vi "AWS Keys Updater(SubVI).vi"(7 "Queue in":refnum<queue>, 8 "error in (no error)":errorcluster) -> ()   [LabVIEW 2019]
doc: "Updates the AWS Access and Secret keys if a properly formatted file is received in the ~/AWS/incoming folder. \n\nThis is to do on-the-fly changes to the AWS credentials (without stopping/restarting MODAQ) and is not a subsitution to valid keys being set in the configurator.\n\nWhy is this necessary? For security purposes, some organizations may time limit AWS keys. It's possible that the AWS keys could expire during a long MODAQ deployment, therefore we provide a way to hot-update the AWS keys without stopping the current MODAQ run. \n\n2021 NREL"
uses:
  Globals and Definitions/System Message.ctl
  Globals and Definitions/Initialization Globals.vi
  Globals and Definitions/RT Globals RD v1.0.vi
  <vilib>/National Instruments/LabVIEW Interface for Amazon S3/LV Interface for Amazon S3.lvlib
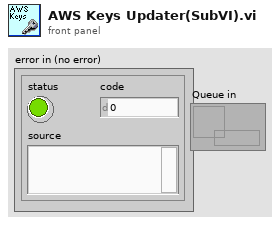
[diagram p1: front panel]
types:
  T1 = typedef "System Message.ctl" = cluster{"Message Tag":string, "Message Body":string, "Snooze Time (s)":dbl, "Snooze Alert?":bool, "Log Event?":bool, "Send Email":i32}
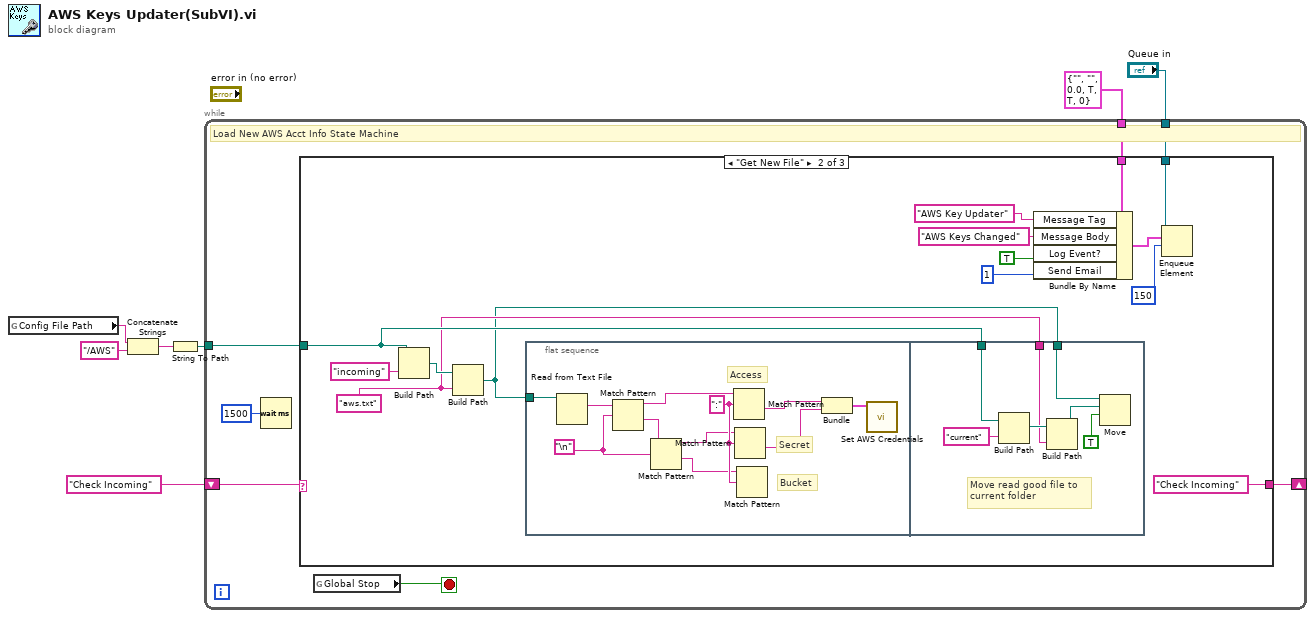
[diagram p0: block diagram]
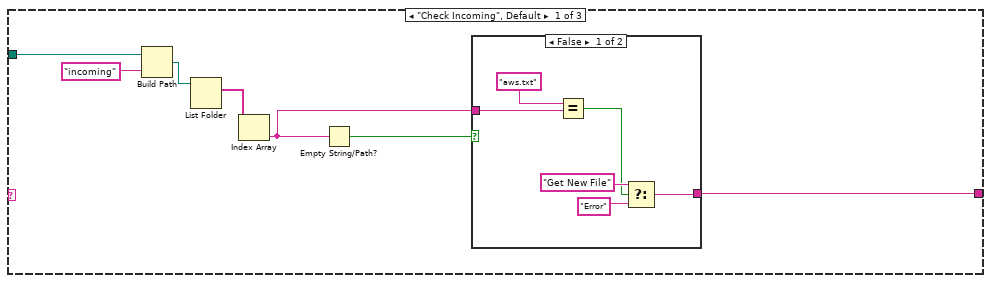
[diagram p2: hidden frame]
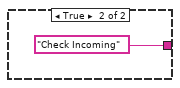
[diagram p3: hidden frame]
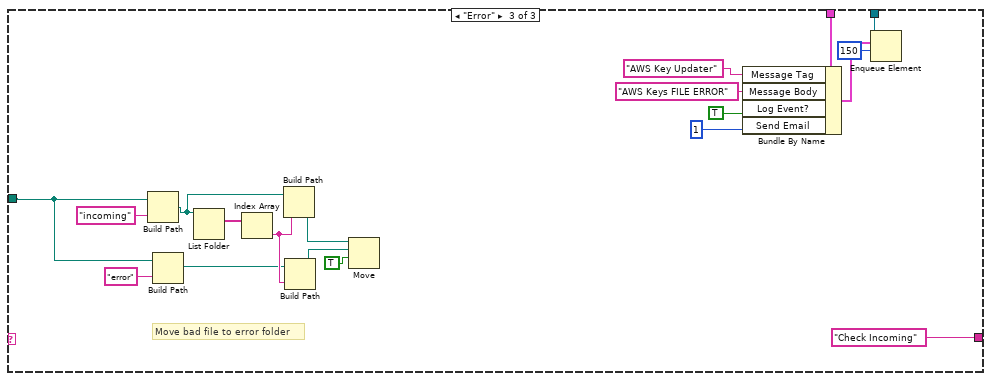
[diagram p4: hidden frame]
diagram:
  n1 = global read "Initialization Globals.vi" "Config File Path"() -> (w4:string)
  n2 = Concatenate Strings(w4, "/AWS" ("string")) -> (w6:string)
  n3 = String To Path(string=w6) -> (path=w7:path)
  n4 = while {
    shift-right: [w13] -> _
    shift-left: "Check Incoming" -> [w11]
    tunnel: w7 -> [w12]
    tunnel: T1 {"Message Tag"="", "Message Body"="", "Snooze Time (s)"=0.0, "Snooze Alert?"=TRUE, "Log Event?"=TRUE, "Send Email"=0} -> [w9]
    tunnel: "Queue in" -> [w8]
    stop <- w10 stop-if-true
    # "Load New AWS Acct Info State Machine"
    n5 = Wait (ms)(milliseconds to wait=u32 1500) -> ()  [unwired: 1 out]
    n6 = case shown="\"Get New File\"" w11 {
      tunnel: [w15 "Check Incoming" "Check Incoming"] -> w13
      tunnel: w12 -> [w16 w40 w73]
      tunnel: w9 -> [_ w32 w64]
      tunnel: w8 -> [_ w31 w63]
      frame "Check Incoming", Default {
        n7 = Build Path(base path=w16, name or relative path="incoming") -> (appended path=w19:path)
        n8 = List Folder(path=w19) -> (filenames=w21:string[])  [unwired: 3 in, 3 out]
        n9 = Index Array(array=w21) -> (element=w17:string)  [unwired: 1 in]
        n10 = Empty String/Path?(string/path=w17) -> (empty?=w18:bool)
        n11 = case shown="False" w18 {
          tunnel: [w22 "Check Incoming"] -> w15
          tunnel: w17 -> [w26 _]
          frame False {
            n12 = Equal?(x="aws.txt", y=w26) -> (x = y?=w23:bool)
            n13 = Select(t="Get New File", s=w23, f="Error") -> (s? t:f=w22:string)
          }
          frame True {
          }
        }
      }
      frame "Get New File" {
        w39 = "aws.txt"
        n14 = Build Path(base path=w40, name or relative path="incoming") -> (appended path=w41:path)
        n15 = Build Path(base path=w41, name or relative path=w39) -> (appended path=w37:path)
        n16 = flat-sequence {
          tunnel: w37 -> [w46]
          tunnel: w40 -> [w57]
          tunnel: w39 -> [w56]
          tunnel: w37 -> [w55]
          frame #0 {
            w49 = ":" ("regular expression")
            w51 = "\n"
            # "Bucket"
            # "Secret"
            # "Access"
            n17 = Read from Text File(file (use dialog)=w46) -> (text=w53:string)  [unwired: 3 in, 3 out]
            n18 = Match Pattern(string=w53, regular expression=w51) -> (before substring=w50:string, after substring=w52:string)  [unwired: 1 in, 2 out]
            n19 = Match Pattern(string=w52, regular expression=w51) -> (before substring=w48:string, after substring=w47:string)  [unwired: 1 in, 2 out]
            n20 = Match Pattern(string=w50, regular expression=w49) -> (after substring=w44:string)  [unwired: 1 in, 3 out]
            n21 = Match Pattern(string=w48, regular expression=w49) -> (after substring=w43:string)  [unwired: 1 in, 3 out]
            n22 = Match Pattern(string=w47, regular expression=w49) -> ()  [unwired: 1 in, 4 out]
            n23 = Bundle(w44, w43) -> (w45:cluster{string, string})  [unwired: 1 in]
            n24 = call <vilib>:"Set AWS Credentials.vi"("AWS Credentials in"=w45) -> ()  [unwired: 10 in, 1 out]
          }
          frame #1 {
            # "Move read good file to\ncurrent folder"
            n25 = Build Path(base path=w57, name or relative path="current") -> (appended path=w59:path)
            n26 = Build Path(base path=w59, name or relative path=w56) -> (appended path=w60:path)
            n27 = Move(source path=w55, 9:TRUE ("overwrite (F)"), 10:w60) -> ()  [unwired: 2 in, 3 out]
          }
        }
        n28 = Bundle By Name(cluster=w32, "Message Tag"="AWS Key Updater", "Message Body"="AWS Keys Changed", "Log Event?"=TRUE, "Send Email"=1) -> (w30:T1)
        n29 = Enqueue Element(queue=w31, element=w30, timeout in ms (-1)=150) -> ()  [unwired: 1 in, 3 out]
      }
      frame "Error" {
        # "Move bad file to error folder"
        n30 = Build Path(base path=w73, name or relative path="incoming") -> (appended path=w76:path)
        n31 = Build Path(base path=w73, name or relative path="error") -> (appended path=w71:path)
        n32 = List Folder(path=w76) -> (filenames=w77:string[])  [unwired: 3 in, 3 out]
        n33 = Index Array(array=w77) -> (element=w72:string)  [unwired: 1 in]
        n34 = Build Path(base path=w76, name or relative path=w72) -> (appended path=w75:path)
        n35 = Build Path(base path=w71, name or relative path=w72) -> (appended path=w70:path)
        n36 = Move(source path=w75, 9:TRUE ("overwrite (F)"), 10:w70) -> ()  [unwired: 2 in, 3 out]
        n37 = Bundle By Name(cluster=w64, "Message Tag"="AWS Key Updater", "Message Body"="AWS Keys FILE ERROR", "Log Event?"=TRUE, "Send Email"=1) -> (w62:T1)
        n38 = Enqueue Element(queue=w63, element=w62, timeout in ms (-1)=150) -> ()  [unwired: 1 in, 3 out]
      }
    }
    n39 = global read "RT Globals RD v1.0.vi" "Global Stop"() -> (w10:bool)
  }
